vi "De-Initialize.vi"(8 "error in":errorcluster, 11 "Messaging Structures":T1) -> (0 "error out":errorcluster)   [LabVIEW 2020, in "Support.lvlib"]
doc: "This VI will close / release all project references (messaging structures, database connection, ...)"
uses:
  Support.lvlib
  Controls/Project Messaging Structures.ctl
  Controls/Project Event Msg.ctl
  Controls/Project Events.ctl
  Error Handler/Controls/Error QMsg.ctl
  Controls/Project Modules.ctl
  Controller/Controls/Controller QMsg.ctl
  Controller/Controller.lvlib
  Error Handler/ErrorHandler.lvlib
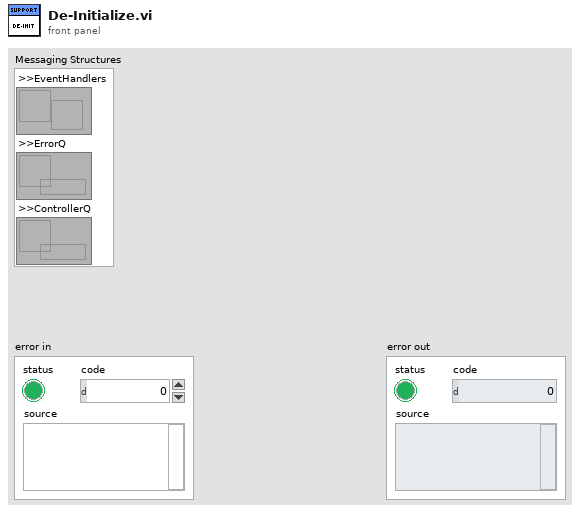
[diagram p1: front panel]
types:
  T1 = typedef "Support.lvlib/Project Messaging Structures.ctl" = cluster{">>EventHandlers":refnum<user-event>, ">>ErrorQ":refnum<queue>, ">>ControllerQ":refnum<queue>}
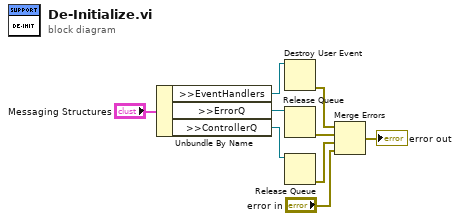
[diagram p0: block diagram]
diagram:
  n1 = Unbundle By Name("Messaging Structures") -> (">>EventHandlers"=w8:refnum<user-event>, ">>ErrorQ"=w7:refnum<queue>, ">>ControllerQ"=w6:refnum<queue>)
  n2 = Destroy User Event(user event=w8) -> (error out=w5:errorcluster)  [unwired: 1 in]
  n3 = Release Queue(queue=w7) -> (error out=w4:errorcluster)  [unwired: 2 in, 2 out]
  n4 = Release Queue(queue=w6) -> (error out=w3:errorcluster)  [unwired: 2 in, 2 out]
  n5 = Merge Errors(w5, w4, w3, "error in") -> (→"error out":errorcluster)
